vi "變數傳進Q的練習.vi"(8 "error in (no error)":errorcluster, 10 "data":T1, 11 "Enum":T2) -> (0 "error out":errorcluster)   [LabVIEW 2019]
uses:
  Ctrl/ModbusCmd.ctl
  Subvi/RobotControlQueueIn.vi
panel:
  out "Holding Registers":u16[](array[numeric])
  out "Sat Coils":bool[](array[boolean])
  out "data 2":T1
  in  "variant 5":variant
  in  "data 3":T1
  out "variant 4":variant
  in  "Data":variant
  out "variant 2":variant
  out "variant":variant
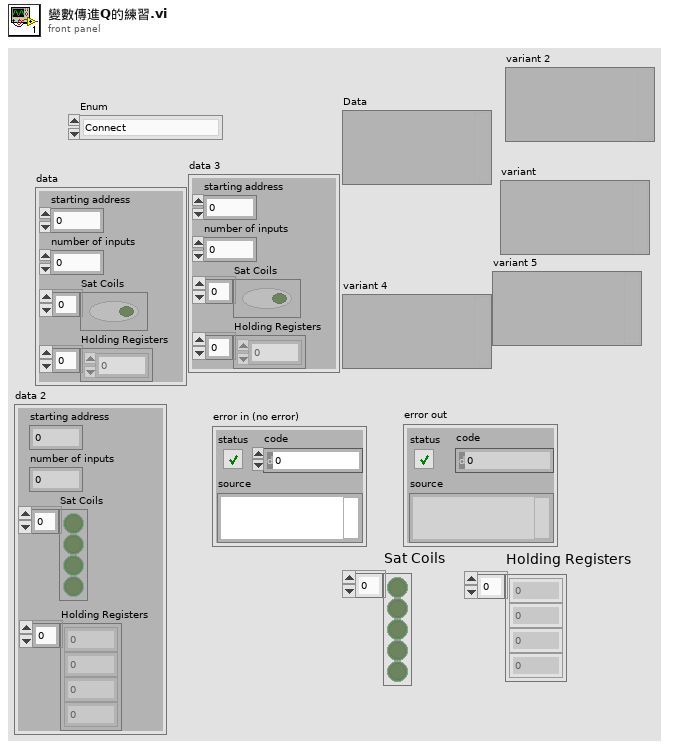
[diagram p1: front panel]
types:
  T1 = cluster{"starting address":u16, "number of inputs":u16, "Sat Coils":bool[], "Holding Registers":u16[]}
  T2 = typedef "ModbusCmd.ctl" = enum16{"Connect", "Disconnect", "Init", "Fetch Basic Objects", "Fetch Input Refisters", "Fetch Discrete Inputs", "Set Coils", "Set Holding Registers", "Write Single Holding", "Exit"}
  T3 = cluster{"starting address":u16, "starting address 2":u16, bool[], "Holding Registers":u16[]}
  T4 = cluster{"starting address":u16, "number of inputs":u16, "Sat Coils":bool[]}
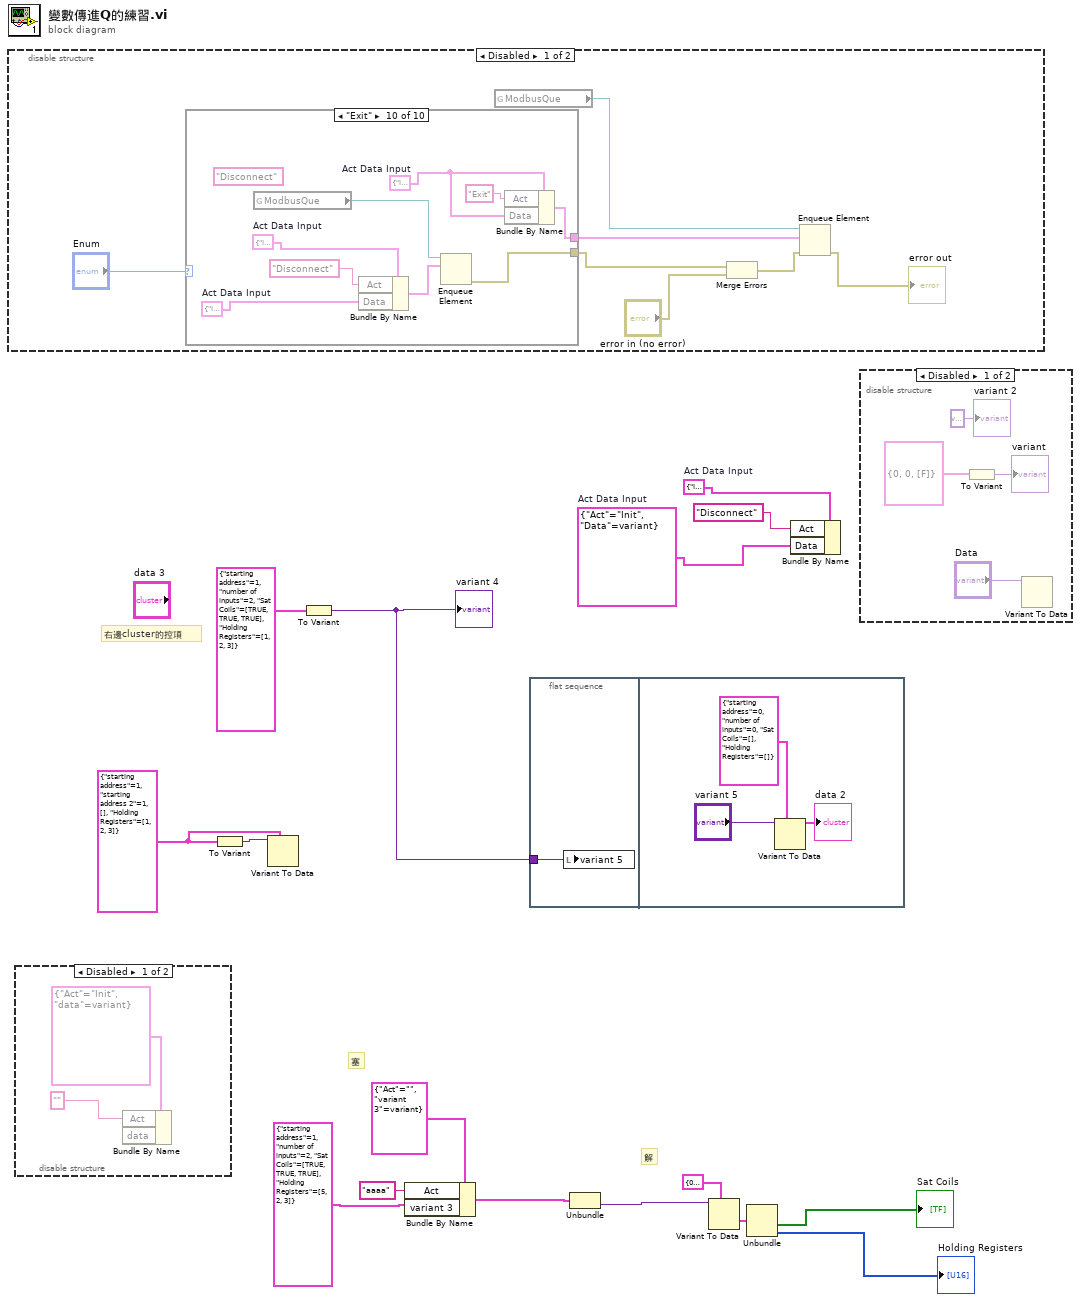
[diagram p0: block diagram]
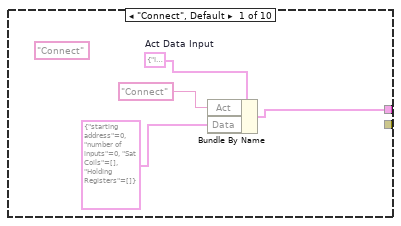
[diagram p2: hidden frame]
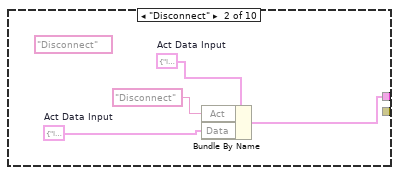
[diagram p3: hidden frame]
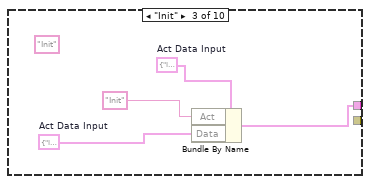
[diagram p4: hidden frame]
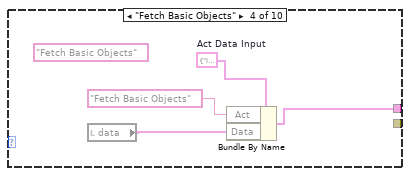
[diagram p5: hidden frame]
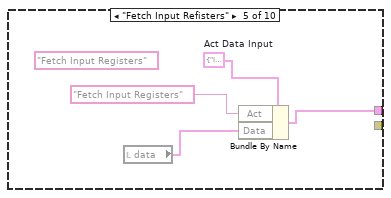
[diagram p6: hidden frame]
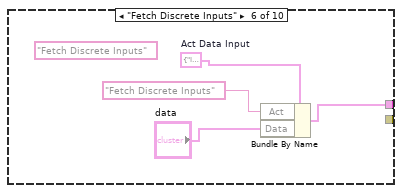
[diagram p7: hidden frame]
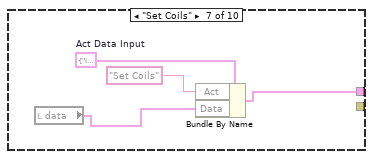
[diagram p8: hidden frame]
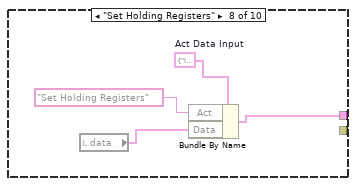
[diagram p9: hidden frame]
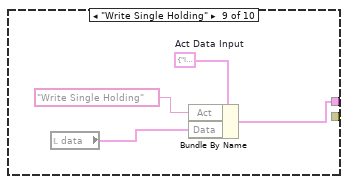
[diagram p10: hidden frame]
diagram:
  w10 = T3 {"starting address"=1, "starting address 2"=1, [], "Holding Registers"=[1, 2, 3]}
  w14 = cluster{"Act":string, "Data":variant} {"Act"="Init", "Data"=variant}  # Act Data Input
  w15 = cluster{"Act":string, "Data":variant} {"Act"="Init", "Data"=variant}  # Act Data Input
  # "塞"
  # "解"
  # "右邊cluster的控項"
  n1 = disable-structure shown="Disabled" {
    frame Disabled {
      n2 = case shown="\"Exit\"" "Enum" {
        tunnel: [w26 w30 w34 w38 w42 w46 w50 w54 w56 w63] -> w18
        tunnel: [_ _ _ _ _ _ _ _ _ w67] -> w20
        frame "Connect", Default {
          w25 = cluster{"Act":string, "Data":variant} {"Act"="Init", "Data"=variant}  # Act Data Input
          (unwired) "Connect" ("element")
          n3 = Bundle By Name(cluster=w25, "Act"="Connect", "Data"=T1 {"starting address"=0, "number of inputs"=0, "Sat Coils"=[], "Holding Registers"=[]} ("data")) -> (w26:cluster{"Act":string, "Data":variant})
        }
        frame "Disconnect" {
          w28 = cluster{"Act":string, "Data":variant} {"Act"="Init", "Data"=variant}  # Act Data Input
          w29 = cluster{"Act":string, "Data":variant} {"Act"="Init", "Data"=variant}  # Act Data Input
          (unwired) "Disconnect" ("element")
          n4 = Bundle By Name(cluster=w29, "Act"="Disconnect", "Data"=w28) -> (w30:cluster{"Act":string, "Data":variant})
        }
        frame "Init" {
          w32 = cluster{"Act":string, "Data":variant} {"Act"="Init", "Data"=variant}  # Act Data Input
          w33 = cluster{"Act":string, "Data":variant} {"Act"="Init", "Data"=variant}  # Act Data Input
          (unwired) "Init" ("element")
          n5 = Bundle By Name(cluster=w33, "Act"="Init", "Data"=w32) -> (w34:cluster{"Act":string, "Data":variant})
        }
        frame "Fetch Basic Objects" {
          w37 = cluster{"Act":string, "Data":variant} {"Act"="Init", "Data"=variant}  # Act Data Input
          (unwired) "Fetch Basic Objects" ("element")
          n6 = local read "data"() -> (w36:T1)
          n7 = Bundle By Name(cluster=w37, "Act"="Fetch Basic Objects", "Data"=w36) -> (w38:cluster{"Act":string, "Data":variant})
        }
        frame "Fetch Input Refisters" {
          w41 = cluster{"Act":string, "Data":variant} {"Act"="Init", "Data"=variant}  # Act Data Input
          (unwired) "Fetch Input Registers" ("element")
          n8 = local read "data"() -> (w40:T1)
          n9 = Bundle By Name(cluster=w41, "Act"="Fetch Input Registers", "Data"=w40) -> (w42:cluster{"Act":string, "Data":variant})
        }
        frame "Fetch Discrete Inputs" {
          w45 = cluster{"Act":string, "Data":variant} {"Act"="Init", "Data"=variant}  # Act Data Input
          (unwired) "Fetch Discrete Inputs" ("element")
          n10 = Bundle By Name(cluster=w45, "Act"="Fetch Discrete Inputs", "Data"="data") -> (w46:cluster{"Act":string, "Data":variant})
        }
        frame "Set Coils" {
          w48 = cluster{"Act":string, "Data":variant} {"Act"="Init", "Data"=variant}  # Act Data Input
          n11 = local read "data"() -> (w49:T1)
          n12 = Bundle By Name(cluster=w48, "Act"="Set Coils", "Data"=w49) -> (w50:cluster{"Act":string, "Data":variant})
        }
        frame "Set Holding Registers" {
          w53 = cluster{"Act":string, "Data":variant} {"Act"="Init", "Data"=variant}  # Act Data Input
          n13 = local read "data"() -> (w52:T1)
          n14 = Bundle By Name(cluster=w53, "Act"="Set Holding Registers", "Data"=w52) -> (w54:cluster{"Act":string, "Data":variant})
        }
        frame "Write Single Holding" {
          w58 = cluster{"Act":string, "Data":variant} {"Act"="Init", "Data"=variant}  # Act Data Input
          n15 = local read "data"() -> (w59:T1)
          n16 = Bundle By Name(cluster=w58, "Act"="Write Single Holding", "Data"=w59) -> (w56:cluster{"Act":string, "Data":variant})
        }
        frame "Exit" {
          w60 = cluster{"Act":string, "Data":variant} {"Act"="Init", "Data"=variant}  # Act Data Input
          w61 = cluster{"Act":string, "Data":variant} {"Act"="Init", "Data"=variant}  # Act Data Input
          w62 = cluster{"Act":string, "Data":variant} {"Act"="Init", "Data"=variant}  # Act Data Input
          (unwired) "Disconnect" ("element")
          n17 = global read "RobotControlQueueIn.vi" "ModbusQue"() -> (w68:refnum<queue>)
          n18 = Bundle By Name(cluster=w61, "Act"="Disconnect", "Data"=w62) -> (w65:cluster{"Act":string, "Data":variant})
          n19 = Enqueue Element(queue=w68, element=w65) -> (error out=w67:errorcluster)  [unwired: 2 in, 2 out]
          n20 = Bundle By Name(cluster=w60, "Act"="Exit" ("element"), "Data"=w60) -> (w63:cluster{"Act":string, "Data":variant})
        }
      }
      n21 = global read "RobotControlQueueIn.vi" "ModbusQue"() -> (w23:refnum<queue>)
      n22 = Merge Errors(w20, "error in (no error)") -> (w19:errorcluster)
      n23 = Enqueue Element(queue=w23, element=w18, error in (no error)=w19) -> (error out=→"error out":errorcluster)  [unwired: 1 in, 2 out]
    }
    frame Enabled {
    }
  }
  n24 = disable-structure shown="Disabled" {
    frame Disabled {
      n25 = Bundle By Name(cluster=cluster{"Act":string, "data":variant} {"Act"="Init", "data"=variant}, "Act"="") -> ()  [unwired: 1 in, 1 out]
    }
    frame Enabled {
    }
  }
  n26 = To Variant(anything=w10) -> (Variant=w11:variant)
  n27 = Variant To Data(type=w10, Variant=w11) -> ()  [unwired: 1 in, 2 out]
  n28 = To Variant(anything=T1 {"starting address"=1, "number of inputs"=2, "Sat Coils"=[TRUE, TRUE, TRUE], "Holding Registers"=[1, 2, 3]} ("data")) -> (Variant=w12:variant)
  "variant 4" <- w12
  n29 = Bundle By Name(cluster=cluster{"Act":string, "variant 3":variant} {"Act"="", "variant 3"=variant}, "Act"="aaaa", "variant 3"=T1 {"starting address"=1, "number of inputs"=2, "Sat Coils"=[TRUE, TRUE, TRUE], "Holding Registers"=[5, 2, 3]} ("data")) -> (w4:cluster{"Act":string, "variant 3":variant})
  n30 = flat-sequence {
    tunnel: w12 -> [w71]
    frame #0 {
      n31 = local write "variant 5"(w71) -> ()
    }
    frame #1 {
      n32 = Variant To Data(type=T1 {"starting address"=0, "number of inputs"=0, "Sat Coils"=[], "Holding Registers"=[]} ("data"), Variant="variant 5") -> (data=→"data 2":T1)  [unwired: 1 in, 1 out]
    }
  }
  n33 = Unbundle "Unbundle"(w4) -> ("variant 3"=w3:variant)  [unwired: 1 out]
  n34 = Variant To Data(type=T1 {"starting address"=0, "number of inputs"=0, "Sat Coils"=[FALSE], "Holding Registers"=[0, 0, 0, 0, 0, 0, 0, 0]} ("output cluster 2"), Variant=w3) -> (data=w5:T1)  [unwired: 1 in, 1 out]
  n35 = Unbundle(w5) -> ("Sat Coils"=→"Sat Coils":bool[], "Holding Registers"=→"Holding Registers":u16[])  [unwired: 2 out]
  n36 = Bundle By Name(cluster=w15, "Act"="Disconnect", "Data"=w14) -> ()  [unwired: 1 out]
  n37 = disable-structure shown="Disabled" {
    frame Disabled {
      n38 = To Variant(anything=T4 {"starting address"=0, "number of inputs"=0, "Sat Coils"=[FALSE]} ("output cluster 2")) -> (Variant=→"variant":variant)
      n39 = Variant To Data(Variant="Data") -> ()  [unwired: 2 in, 2 out]
      "variant 2" <- variant ("variant 2")
    }
    frame Enabled {
    }
  }
